vi "Set Compiler Level.vi"(8 "error in (no error)":errorcluster, 10 "compiler Level (1)":u32=1, 11 "NI_AB_API_DLL in":refnum<class "NI_AB_API_DLL.lvclass">) -> (0 "error out":errorcluster, 3 "NI_AB_API_DLL out":refnum<class "NI_AB_API_DLL.lvclass">)   [LabVIEW 2020, in "NI_AB_API_DLL.lvclass"]
uses:
  <vilib>/AppBuilder/AB_API/DLL/NI_AB_API_DLL.lvclass
  <vilib>/AppBuilder/AB_API/DLL/NI_AB_API_DLL.lvclass/NI_AB_API_DLL.ctl
  <vilib>/AppBuilder/AB_API/Application/NI_AB_API_Application.lvclass
panel:
  # "0: SSE2 optimization disabled\n1: SSE2 optimization enabled"
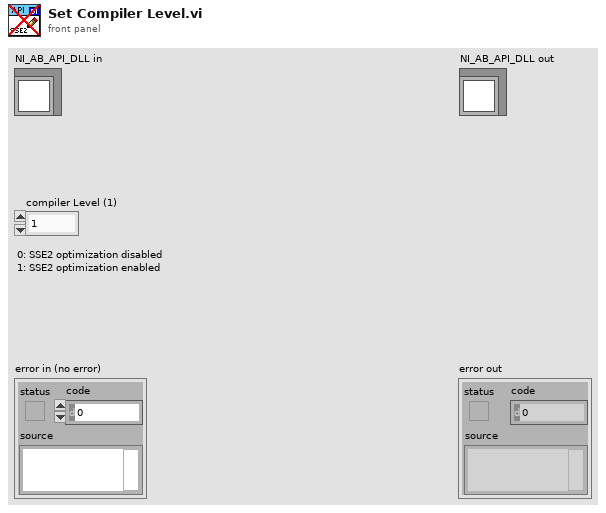
[diagram p1: front panel]
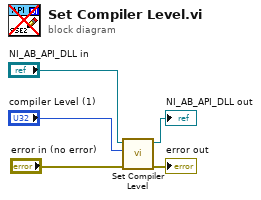
[diagram p0: block diagram]
diagram:
  n1 = call-parent "Set Compiler Level.vi"("error in (no error)"="error in (no error)", "compiler Level (1)"="compiler Level (1)", "NI_AB_API_Build in"="NI_AB_API_DLL in") -> ("error out"=→"error out":errorcluster, "NI_AB_API_Build out"=→"NI_AB_API_DLL out":refnum<class "NI_AB_API_DLL.lvclass">)  [unwired: 7 in]
